vi "InitializeRectanglesByIndex.vi"(8 "error in (no error)":errorcluster, 10 "Index":i32, 11 "Setting Database in":refnum<class "Setting Database.lvclass">) -> (0 "error out":errorcluster, 3 "Setting Database out":refnum<class "Setting Database.lvclass">)   [LabVIEW 2019, in "Setting Database.lvclass"]
uses:
  Setting Database.lvclass
  Setting Database.lvclass/Setting Database.ctl
  <vilib>/Utility/sysdir.llb/Get System Directory.vi
  Rectangle Settings/Rectangle Settings.lvclass
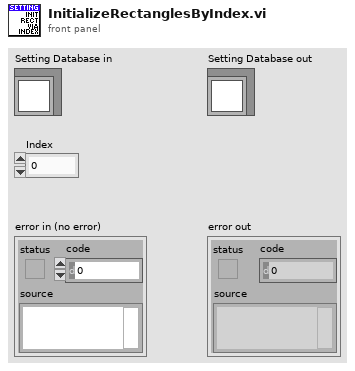
[diagram p1: front panel]
types:
  T1 = cluster{"Path":i32, "Funnel":i32, "Rectangle":i32, "Dot":i32}
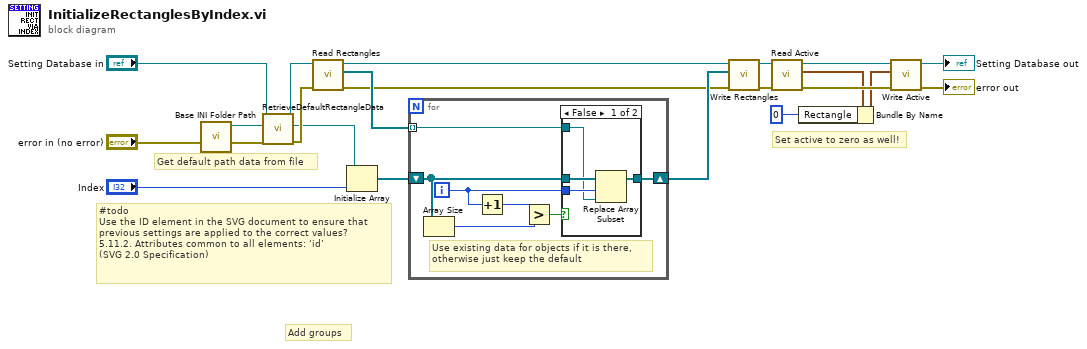
[diagram p0: block diagram]
diagram:
  # "Add groups"
  # "#todo\nUse the ID element in the SVG document to ensure that previous settings are applied to the correct values? \n5.11.2. Attributes common to all elements: ‘id’ \n(SVG 2.0 Specification)"
  # "Get default path data from file"
  # "Set active to zero as well!"
  n1 = call "Base INI Folder Path.vi"() -> ("Base Path"=w1:path)  [unwired: 11 in]
  n2 = call "RetrieveDefaultRectangleData.vi"("error in (no error)"="error in (no error)", "Path"=w1, "Setting Database In"="Setting Database in") -> ("error out"=w10:errorcluster, "Rectangle Settings.lvclass"=w4:refnum<class "Rectangle Settings.lvclass">, "Setting Database Out"=w2:refnum<class "Setting Database.lvclass">)  [unwired: 6 in]
  n3 = call "Read Rectangles.vi"("error in (no error)"=w10, "Setting Database in"=w2) -> ("error out"=w6:errorcluster, "Rectangles"=w11:refnum<class "Rectangle Settings.lvclass">[], "Setting Database out"=w9:refnum<class "Setting Database.lvclass">)  [unwired: 7 in]
  n4 = Initialize Array(w4, "Index") -> (w21:refnum<class "Rectangle Settings.lvclass">[])
  n5 = for {
    tunnel: w11 -> [w28] mode=indexing
    shift-right: [w27] -> w7
    shift-left: w21 -> [w26]
    i -> [w22]
    # "Use existing data for objects if it is there, otherwise just keep the default"
    n6 = Array Size(array=w26) -> (size(s)=w25:i32)
    n7 = Increment(x=w22) -> (x+1=w23:i32)
    n8 = Greater?(x=w23, y=w25) -> (0:w24:bool)
    n9 = case shown="False" w24 {
      tunnel: w28 -> [w29 _]
      tunnel: [w32 w33] -> w27
      tunnel: w26 -> [w31 w33]
      tunnel: w22 -> [w30 _]
      frame False {
        n10 = Replace Array Subset(array=w31, new element=w29, index=w30) -> (w32:refnum<class "Rectangle Settings.lvclass">[])
      }
      frame True {
      }
    }
  }
  n11 = call "Write Rectangles.vi"("error in (no error)"=w6, "Rectangles"=w7, "Setting Database in"=w9) -> ("error out"=w5:errorcluster, "Setting Database out"=w8:refnum<class "Setting Database.lvclass">)  [unwired: 7 in]
  n12 = call "Read Active.vi"("error in (no error)"=w5, "Setting Database in"=w8) -> ("error out"=w19:errorcluster, "Active"=w18:T1, "Setting Database out"=w20:refnum<class "Setting Database.lvclass">)  [unwired: 7 in]
  n13 = Bundle By Name(cluster=w18, "Rectangle"=0 ("Path")) -> (w16:T1)
  n14 = call "Write Active.vi"("error in (no error)"=w19, "Active"=w16, "Setting Database in"=w20) -> ("error out"=→"error out":errorcluster, "Setting Database out"=→"Setting Database out":refnum<class "Setting Database.lvclass">)  [unwired: 7 in]
